vi "SubVI.vi"() -> ()   [LabVIEW 2021]
panel:
  out "Numeric":dbl
  in  "Stop":bool
  out "Gauge":dbl(knob) scale=0.0..200.0
  in  "Vertical Pointer Slide":dbl(slide) scale=0.0..100.0
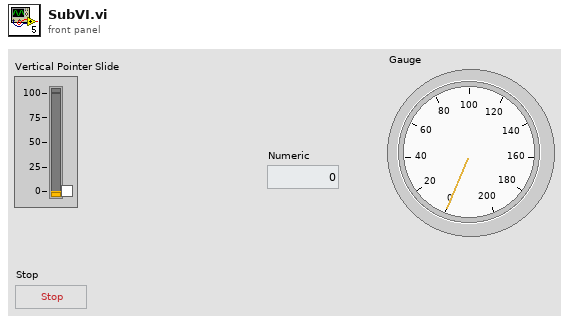
[diagram p1: front panel]
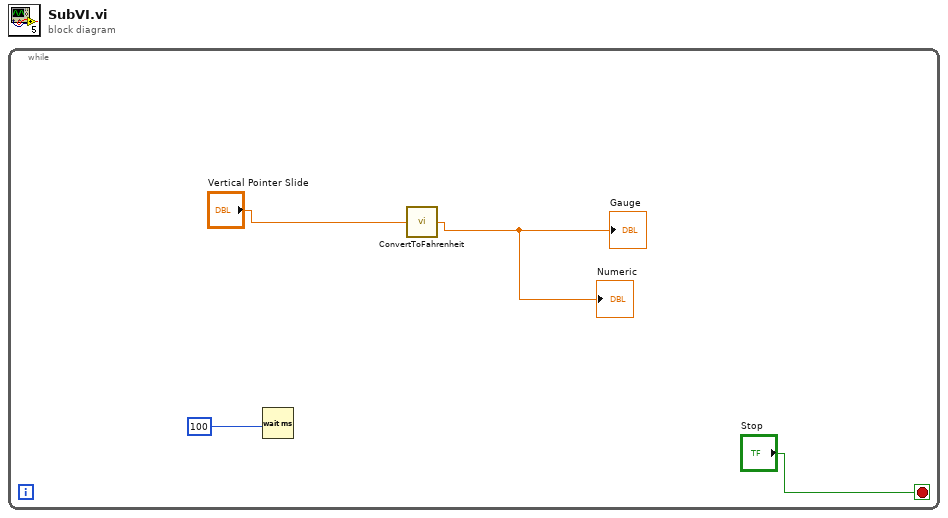
[diagram p0: block diagram]
diagram:
  n1 = while {
    stop <- "Stop" stop-if-true
    n2 = Wait (ms)(milliseconds to wait=u32 100 ("millisecond timer value")) -> ()  [unwired: 1 out]
    n3 = call "ConvertToFahrenheit.vi"("Celcius"="Vertical Pointer Slide") -> ("fahrenheit"=→"Gauge" →"Numeric":dbl)
  }
